vi "OneShot.vi"(0 "button in":bool) -> (7 "Button Pressed":bool)   [LabVIEW 2017]
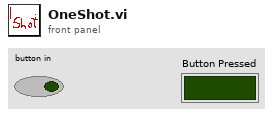
[diagram p1: front panel]
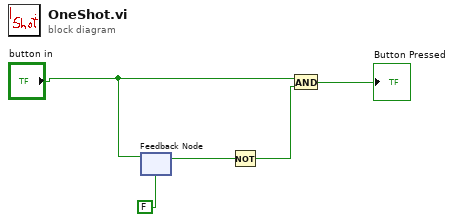
[diagram p0: block diagram]
diagram:
  n1 = feedback-in #1("button in") -> ()
  n2 = feedback #1(FALSE) -> (w2:bool)
  n3 = Not(x=w2) -> (.not. x?=w4:bool)
  n4 = And(x="button in", y=w4) -> (x .and. y?=→"Button Pressed":bool)
